vi "PC_AO_Thermistor Temperature.vi"() -> ()   [LabVIEW 2021]
uses:
  Temperature Thermistor Measurement/Typedefs/Range and Terminal Settings.ctl
  Temperature Thermistor Measurement/Typedefs/Thermistor Parameters.ctl
  Temperature Thermistor Measurement/Typedefs/ABC Parameters.ctl
  Temperature Thermistor Measurement/Typedefs/Beta Parameters.ctl
  Temperature Thermistor Measurement/Typedefs/Specific Channel Settings.ctl
  Temperature Thermistor Measurement/Typedefs/Temperature Thermistor Measurements.ctl
  DC Voltage Generation/DAQ_DC Voltage Generation.lvlib
  Temperature Thermistor Measurement/DAQ_Temperature Thermistor Measurement.lvlib
panel:
  out "error out":errorcluster
  out "Temperature Measurements":T1={"Averaged Temperature (degC)"=[25.01188556420542, 24.99572096279327], "Averaged Temperature (K)"=[298.1618855642054, 298.14572096279323]} {"Averaged Temperature (K)" format="%.2p"; "Averaged Temperature (degC)" format="%.2p"}
  out "Temperature Waveforms":waveform(dbl)[](graph)=[{"t0"=timestamp(3825152236.45778 s since 1904-01-01), "dt"=9.999999999999999e-05, "Y"=array[1000 elements], "attributes"=variant("NI_ChannelName"=variant(string "Dev1/ai2"), "NI_UnitDescription"=variant(string "Deg C"))}, {"t0"=timestamp(3825152236.457791 s since 1904-01-01), "dt"=9.999999999999999e-05, "Y"=array[1000 elements], "attributes"=variant("NI_ChannelName"=variant(string "Dev1/ai4"), "NI_UnitDescription"=variant(string "Deg C"))}]
  in  "Range and Terminal Settings":T2={"Global Settings"={"Min Temp (degC)"=0.0, "Max Temp (degC)"=100.0, "Vex Value (V)"=10.0, "R1 (Ohm)"=5000.0, "Terminal Configuration"=10106, "Thermistor Parameters"={"Type"=enum."Beta", "ABC Parameters"={"A"=0.0, "B"=0.0, "C"=0.0}, "Beta Parameters"={"Beta Value (K)"=3720.0, "R0 (Ohm)"=5000.0}}}, "Specific Channel Settings"=[{"Physical Channel Name"="Dev1/ai2", "Min Temp (degC)"=0.0, "Max Temp (degC)"=100.0, "Vex Value (V) "=10.0, "R1 (Ohm)"=4990.0, "Terminal Configuration"=10106, "Thermistor Parameters"={"Type"=enum."Beta", "ABC Parameters"={"A"=0.0, "B"=0.0, "C"=0.0}, "Beta Parameters"={"Beta Value (K)"=3720.0, "R0 (Ohm)"=5000.0}}}, {"Physical Channel Name"="Dev1/ai4", "Min Temp (degC)"=0.0, "Max Temp (degC)"=100.0, "Vex Value (V) "=10.0, "R1 (Ohm)"=10090.0, "Terminal Configuration"=10083, "Thermistor Parameters"={"Type"=enum."Beta", "ABC Parameters"={"A"=0.0, "B"=0.0, "C"=0.0}, "Beta Parameters"={"Beta Value (K)"=3720.0, "R0 (Ohm)"=10000.0}}}]} {"Specific Channel Settings"."Terminal Configuration" items=["RSE"=10083, "NRSE"=10078, "Differential"=10106]; "Specific Channel Settings"."Thermistor Parameters"."Beta Parameters"."R0 (Ohm)" format="%#.6p"; "Specific Channel Settings"."Thermistor Parameters"."Beta Parameters"."Beta Value (K)" format="%.2f"; "Specific Channel Settings"."Thermistor Parameters"."ABC Parameters"."C" format="%^.6e"; "Specific Channel Settings"."Thermistor Parameters"."ABC Parameters"."B" format="%^.6e"; "Specific Channel Settings"."Thermistor Parameters"."ABC Parameters"."A" format="%^.6e"; "Specific Channel Settings"."R1 (Ohm)" format="%#.2p"; "Specific Channel Settings"."Vex Value (V)" format="%#.2p"; "Specific Channel Settings"."Max Temp (degC)" format="%.2f"; "Specific Channel Settings"."Min Temp (degC)" format="%.2f"; "Global Settings"."Terminal Configuration" items=["RSE"=10083, "NRSE"=10078, "Differential"=10106]; "Global Settings"."Thermistor Parameters"."Beta Parameters"."R0 (Ohm)" format="%#.6p"; "Global Settings"."Thermistor Parameters"."Beta Parameters"."Beta Value (K)" format="%.2f"; "Global Settings"."Thermistor Parameters"."ABC Parameters"."C" format="%^.6e"; "Global Settings"."Thermistor Parameters"."ABC Parameters"."B" format="%^.6e"; "Global Settings"."Thermistor Parameters"."ABC Parameters"."A" format="%^.6e"; "Global Settings"."R1 (Ohm)" format="%#.2p"; "Global Settings"."Vex Value (V)" format="%#.2f"; "Global Settings"."Max Temp (degC)" format="%.2f"; "Global Settings"."Min Temp (degC)" format="%.2f"}
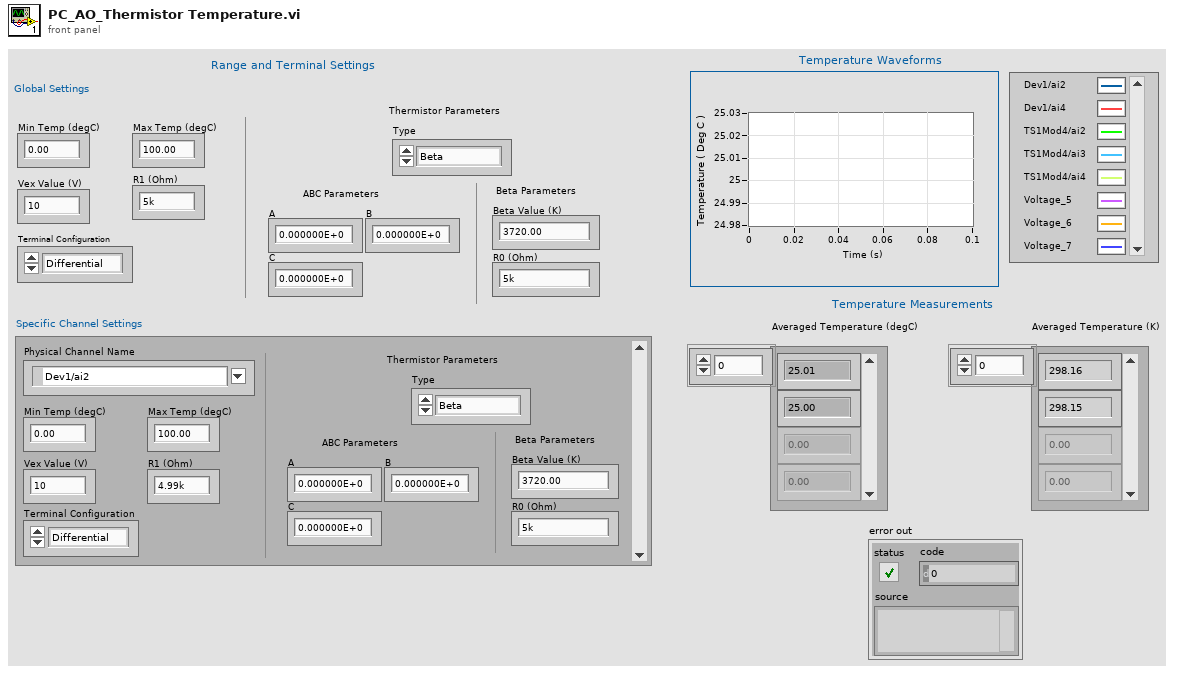
[diagram p1: front panel]
types:
  T1 = typedef "DAQ_Temperature Thermistor Measurement.lvlib/Temperature Thermistor Measurements.ctl" = cluster{"Averaged Temperature (degC)":dbl[], "Averaged Temperature (K)":dbl[]}
  T2 = typedef "DAQ_Temperature Thermistor Measurement.lvlib/Range and Terminal Settings.ctl" = cluster{"Global Settings":cluster{"Min Temp (degC)":dbl, "Max Temp (degC)":dbl, "Vex Value (V)":dbl, "R1 (Ohm)":dbl, "Terminal Configuration":i32, "Thermistor Parameters":T3}, "Specific Channel Settings":T6[]}
  T3 = typedef "DAQ_Temperature Thermistor Measurement.lvlib/Thermistor Parameters.ctl" = cluster{"Type":enum16{"A B C", "Beta"}, "ABC Parameters":T4, "Beta Parameters":T5}
  T4 = typedef "DAQ_Temperature Thermistor Measurement.lvlib/ABC Parameters.ctl" = cluster{"A":dbl, "B":dbl, "C":dbl}
  T5 = typedef "DAQ_Temperature Thermistor Measurement.lvlib/Beta Parameters.ctl" = cluster{"Beta Value (K)":dbl, "R0 (Ohm)":dbl}
  T6 = typedef "DAQ_Temperature Thermistor Measurement.lvlib/Specific Channel Settings.ctl" = cluster{"Physical Channel Name":tag, "Min Temp (degC)":dbl, "Max Temp (degC)":dbl, "Vex Value (V) ":dbl, "R1 (Ohm)":dbl, "Terminal Configuration":i32, "Thermistor Parameters":T3}
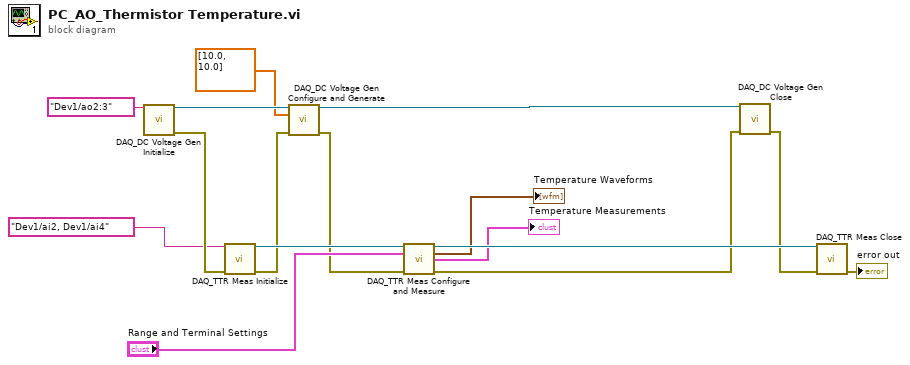
[diagram p0: block diagram]
diagram:
  n1 = call "DAQ_DC Voltage Gen Initialize.vi"("Physical Channels"=tag "Dev1/ao2:3") -> ("DAQmx Task Out"=w3:refnum<k21>, "error out"=w10:errorcluster)  [unwired: 13 in]
  n2 = call "DAQ_TTR Meas Initialize.vi"("Physical Channels"=tag "Dev1/ai2, Dev1/ai4", "error in"=w10) -> ("DAQmx Task Out"=w16:refnum<k21>, "error out"=w9:errorcluster)  [unwired: 12 in]
  n3 = call "DAQ_DC Voltage Gen Configure and Generate.vi"("DAQmx Task In"=w3, "Output Voltages (V)"=dbl[] [10.0, 10.0], "error in"=w9) -> ("DAQmx Task Out"=w2:refnum<k21>, "error out"=w8:errorcluster)  [unwired: 11 in]
  n4 = call "DAQ_TTR Meas Configure and Measure.vi"("DAQmx Task In"=w16, "Range and Terminal Settings"="Range and Terminal Settings", "error in"=w8) -> ("DAQmx Task Out"=w15:refnum<k21>, "Temperature Waveforms"=→"Temperature Waveforms":waveform(dbl)[], "Temperature Measurements"=→"Temperature Measurements":T1, "error out"=w7:errorcluster)  [unwired: 8 in, 1 out]
  n5 = call "DAQ_DC Voltage Gen Close.vi"("DAQmx Task In"=w2, "error in"=w7) -> ("error out"=w6:errorcluster)  [unwired: 13 in]
  n6 = call "DAQ_TTR Meas Close.vi"("DAQmx Task In"=w15, "error in"=w6) -> ("error out"=→"error out":errorcluster)  [unwired: 13 in]
